vi "JDP-JSON Test Marshall-Unmarshall.vi"() -> ()   [LabVIEW 2019]
uses:
  Test Cluster.ctl
  source/Serializer.JDP-JSON.lvclass
  C:/Program Files (x86)/National Instruments/LabVIEW 2019/vi.lib/LabVIEW Open Source Project/OpenSerializer/Serializer/Serializer.lvclass
  source/Serializer.JDP-JSON.lvclass/Serializer.JDP-JSON.ctl
  source/Write Enable LV Extensions.vi
  source/Write Pretty Print.vi
  <vilib>/LabVIEW Open Source Project/OpenSerializer/Serializer/Serializer.lvclass
  <vilib>/JDP Science/JSONtext/JSONtext.lvlib
panel:
  out "error out":errorcluster
  out "Pass?":bool
  out "Data Cluster out":T1={"Top-Level"={"Boolean"=FALSE, "String"="", "Path"=path "", "Numeric"=0.0, "Enum"=enum."Item0", "Array"=[], "Sub-Cluster"={"Numeric"=0.0, "Boolean"=FALSE, "Empty String"=""}, "Multi-Line String"=""}} {"Top-Level"."Numeric" format="%#_10g"}
  out "JSON String":string
  in  "Pretty Print":bool=TRUE
  in  "Enable LV Extensions":bool=TRUE
  in  "Data Cluster in":T1={"Top-Level"={"Boolean"=FALSE, "String"="Another test string", "Path"=path "C:/Windows", "Numeric"=4.0, "Enum"=enum."Item0", "Array"=[0.0, 1.0, 2.0, 3.0, 4.0, 5.0, 6.0], "Sub-Cluster"={"Numeric"=0.0, "Boolean"=TRUE, "Empty String"="Test String Here"}, "Multi-Line String"="Test String Here\nLine2\nLine3"}} {"Top-Level"."Numeric" format="%#_10g"}
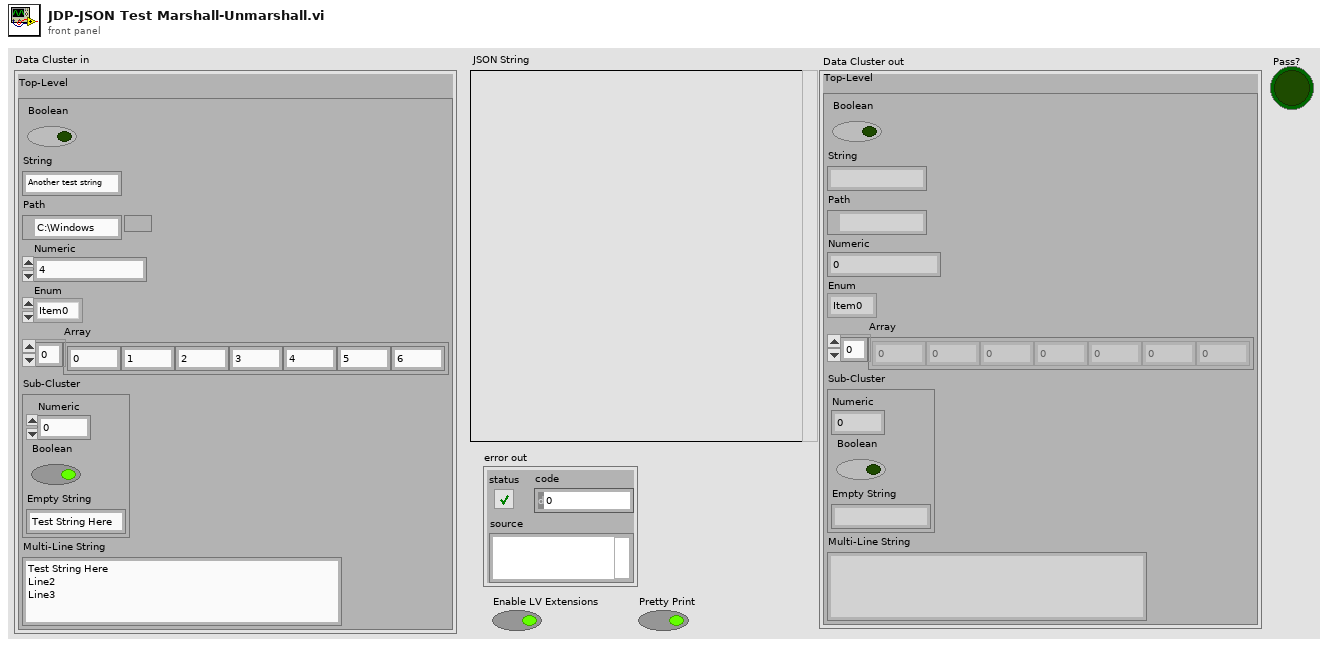
[diagram p1: front panel]
types:
  T1 = typedef "Test Cluster.ctl" = cluster{"Top-Level":cluster{"Boolean":bool, "String":string, "Path":path, "Numeric":dbl, "Enum":enum16{"Item0", "Item1"}, "Array":dbl[], "Sub-Cluster":cluster{"Numeric":dbl, "Boolean":bool, "Empty String":string}, "Multi-Line String":string}}
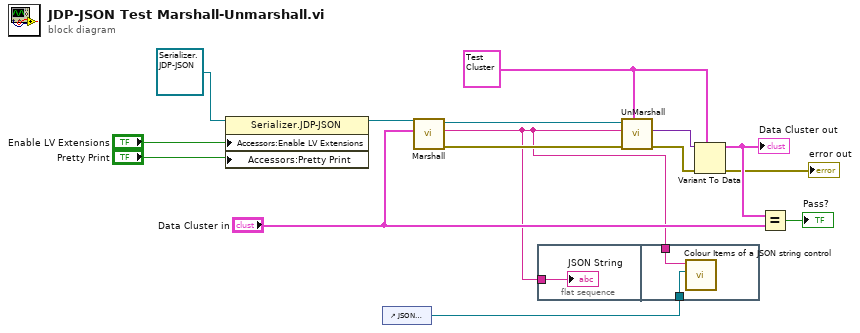
[diagram p0: block diagram]
diagram:
  w7 = T1 {"Top-Level"={"Boolean"=FALSE, "String"="", "Path"=path "", "Numeric"=0.0, "Enum"=enum."Item0", "Array"=[], "Sub-Cluster"={"Numeric"=0.0, "Boolean"=FALSE, "Empty String"=""}, "Multi-Line String"="Test String Here\nLine2\nLine3"}} ("Cluster")
  n1 = property class="Serializer.JDP-JSON"(reference=refnum<class "Serializer.JDP-JSON.lvclass"> refnum ("OpenSerializer.JDP-JSON.lvlib:Serializer.JDP-JSON.lvclass"), "Accessors:Enable LV Extensions"="Enable LV Extensions", "Accessors:Pretty Print"="Pretty Print") -> (reference out=w10:refnum<class "Serializer.JDP-JSON.lvclass">)  [unwired: 1 in, 1 out]
  n2 = control-ref of="JSON String"() -> (w3:refnum<vi>)
  n3 = call <vilib>:"Marshall.vi"("Variant"="Data Cluster in", "Serializer in"=w10) -> ("error out"=w15:errorcluster, "String"=w2:string, "Serializer out"=w14:refnum<class "Serializer.JDP-JSON.lvclass">)  [unwired: 7 in]
  n4 = flat-sequence {
    tunnel: w2 -> [w16]
    tunnel: w3 -> [w18]
    tunnel: w2 -> [w17]
    frame #0 {
      "JSON String" <- w16
    }
    frame #1 {
      n5 = call <vilib>:"Colour Items of a JSON string control.vi"("String Control"=w18, "JSON"=w17) -> ()  [unwired: 10 in]
    }
  }
  n6 = call <vilib>:"UnMarshall.vi"("Type"=w7, "error in (no error)"=w15, "String"=w2, "Serializer in"=w14) -> ("error out"=w9:errorcluster, "Variant"=w8:variant)  [unwired: 5 in, 1 out]
  n7 = Variant To Data(error in=w9, type=w7, Variant=w8) -> (data=w6:T1, error out=→"error out":errorcluster)
  "Data Cluster out" <- w6
  n8 = Equal?(x=w6, y="Data Cluster in") -> (x = y?=→"Pass?":bool)
